vi "Motor TF.vi"(9 "CereInput":dbl, 11 "Vel ref":dbl) -> (0 "PD[n]":dbl, 1 "EC[n]":dbl, 2 "e[n]":dbl, 3 "Vel[n]":dbl)   [LabVIEW 2013]
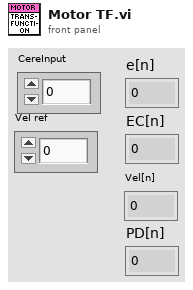
[diagram p1: front panel]
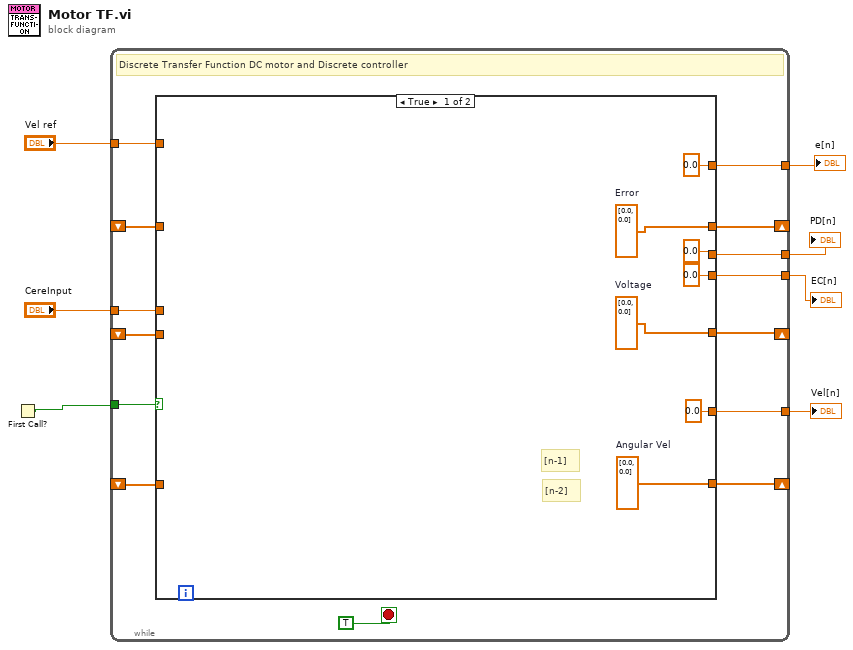
[diagram p0: block diagram]
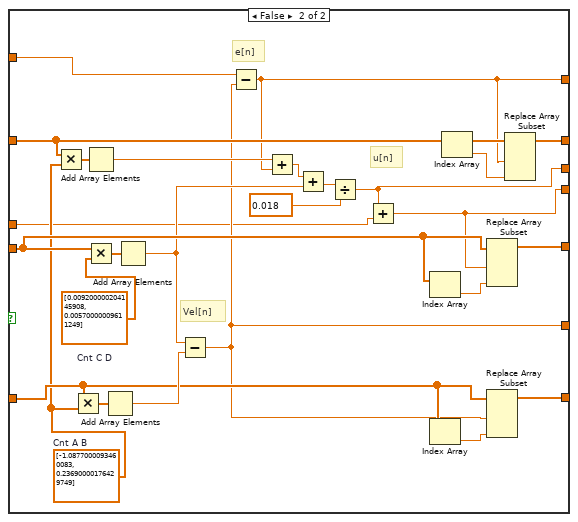
[diagram p2: hidden frame]
diagram:
  n1 = First Call?() -> (First Call?: T/F=w1:bool)
  n2 = while {
    shift-right: [w17] -> _
    shift-left: _ -> [w18]
    shift-right: [w19] -> _
    shift-left: _ -> [w20]
    shift-right: [w16] -> _
    shift-left: _ -> [w15]
    tunnel: "Vel ref" -> [w14]
    tunnel: w1 -> [w13]
    tunnel: [w12] -> w6
    tunnel: [w11] -> w5
    tunnel: [w10] -> w3
    tunnel: "CereInput" -> [w9]
    tunnel: [w8] -> w2
    stop <- TRUE ("stop") stop-if-true
    # "Discrete Transfer Function DC motor and Discrete controller"
    n3 = case shown="True" w13 {
      tunnel: w20 -> [_ w51]
      tunnel: [w27 w49] -> w19
      tunnel: w18 -> [_ w47]
      tunnel: [w26 w46] -> w17
      tunnel: [w28 w44] -> w16
      tunnel: w15 -> [_ w43]
      tunnel: w14 -> [_ w36]
      tunnel: [0.0 w33] -> w12
      tunnel: [0.0 w32] -> w11
      tunnel: [0.0 w30] -> w10
      tunnel: w9 -> [_ w31]
      tunnel: [0.0 w29] -> w8
      frame True {
        w26 = dbl[] [0.0, 0.0]  # Angular Vel
        w27 = dbl[] [0.0, 0.0]  # Voltage
        w28 = dbl[] [0.0, 0.0]  # Error
        # "[n-2]"
        # "[n-1]"
      }
      frame False {
        w34 = dbl[] [0.009200000204145908, 0.00570000009611249]  # Cnt C D
        w35 = dbl[] [-1.0877000093460083, 0.23690000176429749]  # Cnt A B
        # "u[n]"
        # "e[n]"
        # "Vel[n]"
        n4 = Multiply(x=w43, y=w35) -> (x*y=w42:dbl[])
        n5 = Multiply(x=w47, y=w35) -> (x*y=w53:dbl[])
        n6 = Add Array Elements(numeric array=w42) -> (sum=w40:dbl)
        n7 = Multiply(x=w51, y=w34) -> (x*y=w54:dbl[])
        n8 = Add Array Elements(numeric array=w53) -> (sum=w52:dbl)
        n9 = Add Array Elements(numeric array=w54) -> (sum=w39:dbl)
        n10 = Subtract(x=w39, y=w52) -> (x-y=w33:dbl)
        n11 = Subtract(x=w36, y=w33) -> (x-y=w32:dbl)
        n12 = Add(x=w40, y=w32) -> (x+y=w41:dbl)
        n13 = Add(x=w41, y=w39) -> (x+y=w38:dbl)
        n14 = Divide(x=w38, y=0.018) -> (x/y=w29:dbl)
        n15 = Add(x=w29, y=w31) -> (x+y=w30:dbl)
        n16 = Index Array(array=w51) -> (element=w50:dbl)  [unwired: 1 in]
        n17 = Index Array(array=w47) -> (element=w48:dbl)  [unwired: 1 in]
        n18 = Index Array(array=w43) -> (element=w45:dbl)  [unwired: 1 in]
        n19 = Replace Array Subset(array=w51, new element #1=w30, new element #2=w50) -> (w49:dbl[])  [unwired: 2 in]
        n20 = Replace Array Subset(array=w47, new element #1=w33, new element #2=w48) -> (w46:dbl[])  [unwired: 2 in]
        n21 = Replace Array Subset(array=w43, new element #1=w32, new element #2=w45) -> (w44:dbl[])  [unwired: 2 in]
      }
    }
  }
  "Vel[n]" <- w6
  "e[n]" <- w5
  "EC[n]" <- w3
  "PD[n]" <- w2
